vi "校准流程.vi"(0 "校准模式":T3(ring), 5 "参数下拉列表":u16(ring) items=["总氮"=1, "总磷"=2], 7 "测量模式":T1(ring), 9 "量程下拉列表":enum16{"低量程", "高量程"}(ring), 11 "曲线模型":T2={"标液浓度1"=0.0, "测量吸光度1"=0.0, "样品1启用"=FALSE, "标液浓度2"=0.0, "测量吸光度2"=0.0, "样品2启用"=FALSE, "标液浓度3"=0.0, "测量吸光度3"=0.0, "样品3启用"=FALSE, "标液浓度4"=0.0, "测量吸光度4"=0.0, "样品4启用"=FALSE, "标液浓度5"=0.0, "测量吸光度5"=0.0, "样品5启用"=FALSE, "模型"=enum."线性", "精度"=4.0, "XY图"=[], "拟合公式"="", "r^2"=0.0, "标样一校准时间"=timestamp(0 s since 1904-01-01), "标样二校准时间"=timestamp(0 s since 1904-01-01), "标样三校准时间"=timestamp(0 s since 1904-01-01), "标样四校准时间"=timestamp(0 s since 1904-01-01), "标样五校准时间"=timestamp(0 s since 1904-01-01), "二次方程"={"c"=0.0, "x"=0.0, "x^2"=0.0}, "标定时间"=timestamp(0 s since 1904-01-01)} {"标定时间" format="%<%m/%d/%y %H:%M:%S>T"; "标样五校准时间" format="%<%m/%d/%y %H:%M:%S>T"; "标样四校准时间" format="%<%m/%d/%y %H:%M:%S>T"; "标样三校准时间" format="%<%m/%d/%y %H:%M:%S>T"; "标样二校准时间" format="%<%m/%d/%y %H:%M:%S>T"; "标样一校准时间" format="%<%m/%d/%y %H:%M:%S>T"; "r^2" format="%.7f"; "测量吸光度5" format="%#.6f"; "测量吸光度4" format="%#.6f"; "测量吸光度3" format="%#.6f"; "测量吸光度2" format="%#.6f"; "测量吸光度1" format="%#.6f"}) -> ()   [LabVIEW 2016, in "斯坦道CODCr.lvlib"]
panel:
  out "输出簇":cluster{"数据时间":timestamp, "X值":sgl}
  # "校准时间"
  # "标液浓度"
  # "吸光值显示"
  # "标液一"
  # "标液二"
  # "标液三"
  # "零点"
  # "跨度"
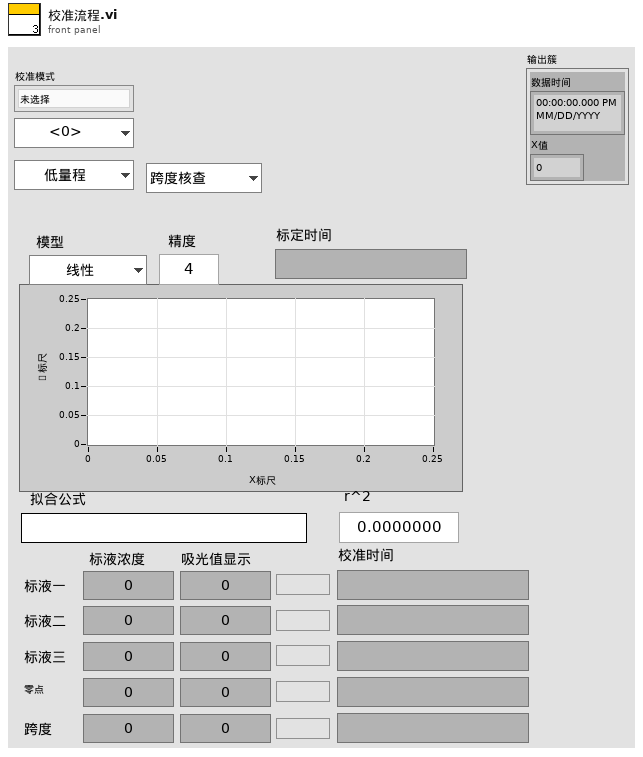
[diagram p1: front panel]
types:
  T1 = enum16{"跨度核查", "水样测量", "零点核查", "标样核查", "加标回收", "快捷测试", "空白校准", "标样校准"}
  T2 = cluster{"标液浓度1":dbl, "测量吸光度1":dbl, "样品1启用":bool, "标液浓度2":dbl, "测量吸光度2":dbl, "样品2启用":bool, "标液浓度3":dbl, "测量吸光度3":dbl, "样品3启用":bool, "标液浓度4":dbl, "测量吸光度4":dbl, "样品4启用":bool, "标液浓度5":dbl, "测量吸光度5":dbl, "样品5启用":bool, "模型":enum32{"线性", "多项式"}, "精度":dbl, "XY图":cluster{"X Values":dbl[], "Y Values":dbl[]}[], "拟合公式":string, "r^2":dbl, "标样一校准时间":timestamp, "标样二校准时间":timestamp, "标样三校准时间":timestamp, "标样四校准时间":timestamp, "标样五校准时间":timestamp, "二次方程":cluster{"c":dbl, "x":dbl, "x^2":dbl}, "标定时间":timestamp}
  T3 = enum32{"未选择", "空白校准", "标样校准", "标样核查", "零点核查", "跨度核查"}
  T4 = enum16{"初始化", "校准启动", "校准运行中", "测试结束", "获取校准数据", "填充校准数据", "流程结束"}
  T5 = cluster{"站号":u16, "量程切换":enum32{"H", "L", "AUTO"}, "控制命令":enum16{"启动测量", "标样核查", "零点核查", "跨度核查", "空白测试", "平行样测试", "加标回收", "空白校准", "标样校准", "初始化（清洗）", "停止测试", "仪器重启", "校时", "模式设置", "测量间隔设置"}, "模式设置":enum16{"待机", "连续模式", "周期模式", "定点模式", "受控模式", "手动模式"}, "测量间隔":u16}
  T6 = enum16{"启动测量", "标样核查", "零点核查", "跨度核查", "空白测试", "平行样测试", "加标回收", "空白校准", "标样校准", "初始化（清洗）", "停止测试", "仪器重启", "校时", "模式设置", "测量间隔设置"}
  T7 = cluster{"因子编码":u32, "单位":u16, "标样参考值":sgl, "水样数据时间":timestamp, "水样实测值":sgl, "水样数据标识":string, "标样数据时间":timestamp, "标样实测值":sgl, "标样数据标识":string, "空白数据时间":timestamp, "空白实测值":sgl, "空白数据标识":string, "零点核查数据时间":timestamp, "零点核查实测值":sgl, "零点核查数据标识":string, "跨度核查数据时间":timestamp, "跨度核查实测值":sgl, "跨度核查数据标识":string, "加标回收数据时间":timestamp, "加标回收实测值":sgl, "加标回收数据标识":string, "平行样数据时间":timestamp, "平行样实测值":sgl, "平行样数据标识":string, "F0":sgl, "F1":sgl, "F2":sgl, "F3":sgl, "F4":sgl, "F5":sgl, "F6":sgl, "F7":sgl, "温度":sgl, "湿度":sgl, "X值":sgl, "fidrange":u16}
  T8 = cluster{"系统时间":timestamp, "工作状态":u16, "测量模式":enum16{"待机", "连续模式", "周期模式", "定点模式", "受控模式", "手动模式"}, "告警代码":u16, "故障代码":u16, "日志代码":u16, "软件版本":u16, "F0":sgl, "F1":sgl, "F2":sgl, "F3":sgl, "T":sgl, "H":sgl, "id":u16, "flowid":u16, "量程":u16, "总磷控温温度1":sgl, "营养盐控温温度2":sgl, "ADC":sgl}
  T9 = cluster{"标液浓度1":dbl, "测量吸光度1":dbl, "样品1启用":bool, "标液浓度2":dbl, "测量吸光度2":dbl, "样品2启用":bool, "标液浓度3":dbl, "测量吸光度3":dbl, "样品3启用":bool, "标液浓度4":dbl, "测量吸光度4":dbl, "样品4启用":bool, "标液浓度5":dbl, "测量吸光度5":dbl, "样品5启用":bool, "模型":enum32{"线性", "多项式"}, "精度":dbl, "XY图":cluster{"X Values":dbl[], "Y Values":dbl[]}[], "拟合公式":string, "r^2":dbl, "标样一校准时间":timestamp, "标样二校准时间":timestamp, "标样三校准时间":timestamp, "标样四校准时间":timestamp, "标样五校准时间":timestamp, "二次方程":cluster{"c":dbl, "x":dbl, "x^2":dbl}, "标定时间":timestamp}[][]
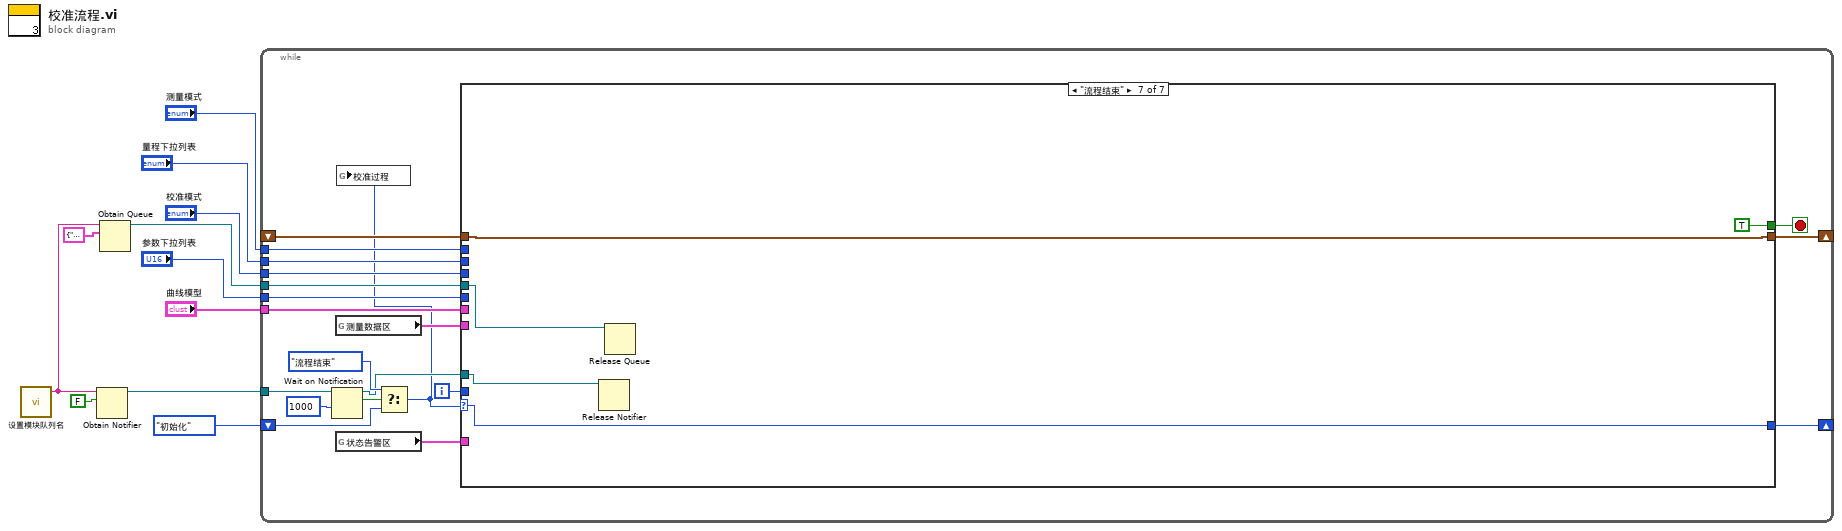
[diagram p0: block diagram]
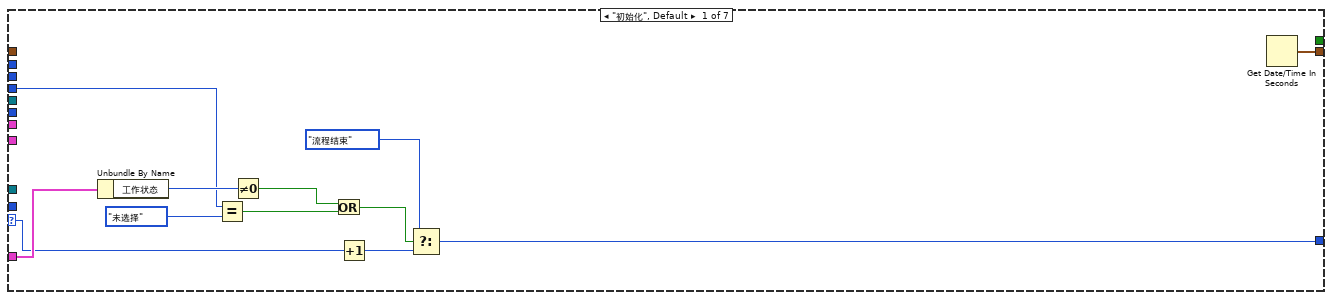
[diagram p2: hidden frame]
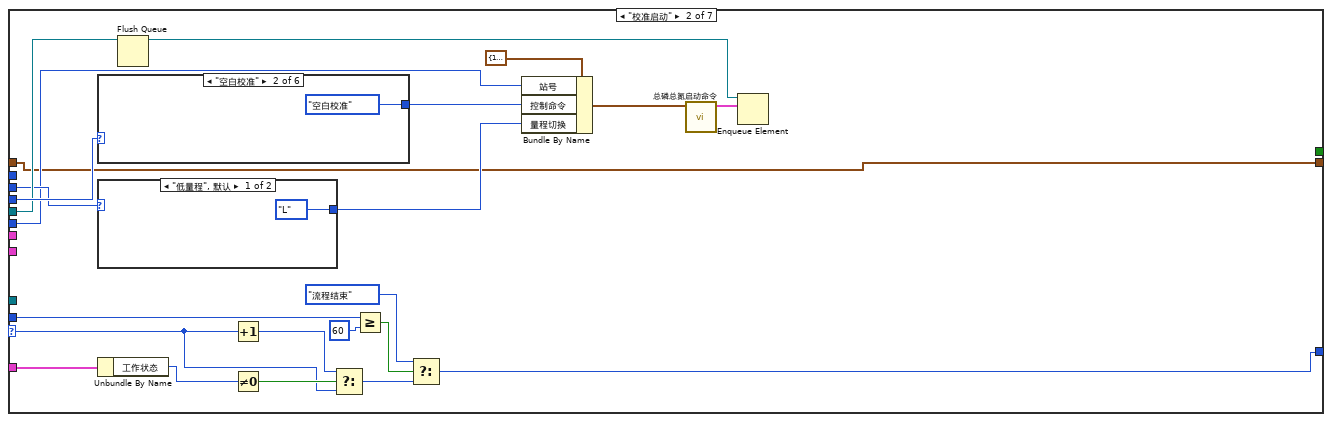
[diagram p3: hidden frame]
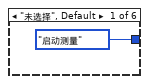
[diagram p4: hidden frame]
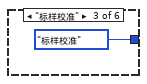
[diagram p5: hidden frame]
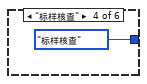
[diagram p6: hidden frame]
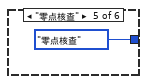
[diagram p7: hidden frame]
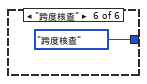
[diagram p8: hidden frame]
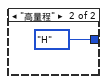
[diagram p9: hidden frame]
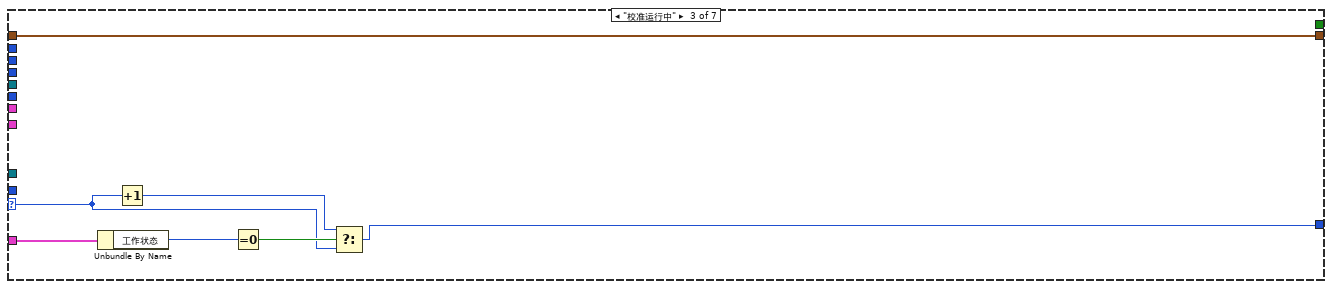
[diagram p10: hidden frame]
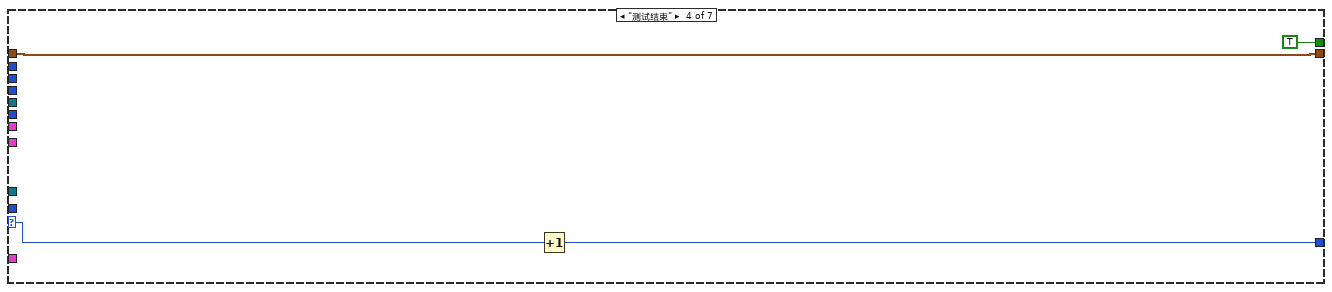
[diagram p11: hidden frame]
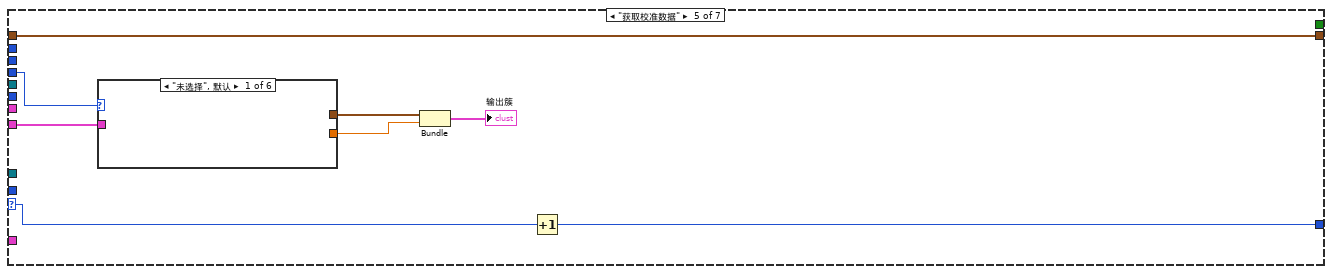
[diagram p12: hidden frame]
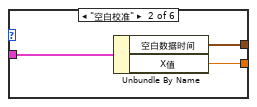
[diagram p13: hidden frame]
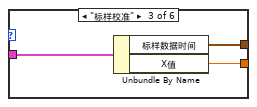
[diagram p14: hidden frame]
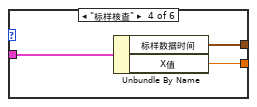
[diagram p15: hidden frame]
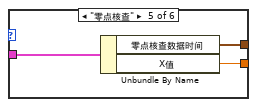
[diagram p16: hidden frame]
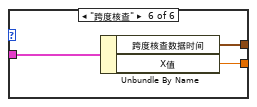
[diagram p17: hidden frame]
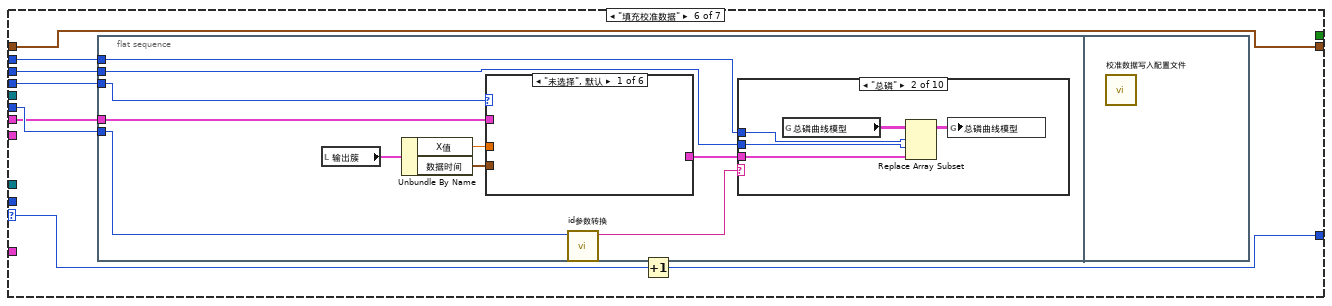
[diagram p18: hidden frame]
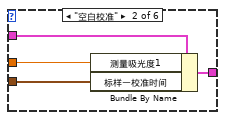
[diagram p19: hidden frame]
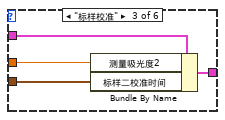
[diagram p20: hidden frame]
diagram:
  n1 = call "设置模块队列名.vi"() -> ("Msg"=w2:string)  [unwired: 5 in]
  n2 = Obtain Notifier(name (unnamed)=w2, notification data type=FALSE) -> (notifier out=w1:refnum<notifier>)  [unwired: 2 in, 2 out]
  n3 = Obtain Queue(name (unnamed)=w2, element data type=cluster{"命令":string, "data":variant} {"命令"="", "data"=variant}) -> (queue out=w8:refnum<queue>)  [unwired: 3 in, 2 out]
  n4 = while {
    tunnel: "校准模式" -> [w30]
    shift-right: [w28] -> _
    shift-left: T4."初始化" ("枚举") -> [w15]
    tunnel: w8 -> [w31]
    tunnel: "量程下拉列表" -> [w27]
    tunnel: "参数下拉列表" -> [w26]
    shift-right: [w25] -> _
    shift-left: _ -> [w24]
    tunnel: "曲线模型" -> [w21]
    tunnel: "测量模式" -> [w20]
    tunnel: w1 -> [w18]
    i -> [w19]
    stop <- w29 stop-if-true
    n5 = Wait on Notification(notifier=w18, timeout in ms (-1)=1000 ("超时毫秒(-1)")) -> (notifier out=w13:refnum<notifier>, notification=w16:bool)  [unwired: 2 in, 2 out]
    n6 = global read "VAR总磷总氮全局变量.vi" "测量数据区"() -> (w23:T7)
    n7 = global read "VAR总磷总氮全局变量.vi" "状态告警区"() -> (w22:T8)
    n8 = Select(t=T4."流程结束", s=w16, f=w15) -> (s? t:f=w12:T4)
    n9 = global write "VAR总磷总氮全局变量.vi" "校准过程"(w12) -> ()
    n10 = case shown="\"流程结束\"" w12 {
      selector: w12 -> [w39 w51 w79 w84 w92 w115 w194]
      tunnel: w31 -> [_ w58 _ _ _ _ w192]
      tunnel: w30 -> [w35 w59 _ _ w89 w109 _]
      tunnel: [_ _ _ TRUE _ _ TRUE] -> w29
      tunnel: [w37 w45 w77 w81 w85 w108 w194] -> w28
      tunnel: w27 -> [_ w57 _ _ _ w112 _]
      tunnel: w26 -> [_ w56 _ _ _ w113 _]
      tunnel: w22 -> [w42 w54 w75 _ _ _ _]
      tunnel: [w43 w55 w76 w83 w91 w114 w193] -> w25
      tunnel: w24 -> [_ w55 w76 w83 w91 w114 w193]
      tunnel: w23 -> [_ _ _ _ w90 _ _]
      tunnel: w21 -> [_ _ _ _ _ w111 _]
      tunnel: w20 -> [_ _ _ _ _ w110 _]
      tunnel: w19 -> [_ w49 _ _ _ _ _]
      tunnel: w13 -> [_ _ _ _ _ _ w191]
      frame "初始化", Default {
        n11 = Unbundle By Name(w42) -> ("工作状态"=w41:u16)
        n12 = Equal?(x=w35, y=T3."未选择") -> (x = y?=w32:bool)
        n13 = Not Equal To 0?(x=w41) -> (x != 0?=w40:bool)
        n14 = Or(x=w40, y=w32) -> (x .or. y?=w33:bool)
        n15 = Increment(x=w39) -> (x+1=w38:T4)
        n16 = Select(t=T4."流程结束", s=w33, f=w38) -> (s? t:f=w37:T4)
        n17 = Get Date/Time In Seconds() -> (seconds since 1Jan1904=w43:timestamp)
      }
      frame "校准启动" {
        n18 = case shown="\"空白校准\"" w59 {
          tunnel: [T6."启动测量" ("控制命令") T6."空白校准" ("控制命令") T6."标样校准" ("控制命令") T6."标样核查" ("控制命令") T6."零点核查" ("控制命令") T6."跨度核查" ("控制命令")] -> w65
          frame "未选择", Default {
          }
          frame "空白校准" {
          }
          frame "标样校准" {
          }
          frame "标样核查" {
          }
          frame "零点核查" {
          }
          frame "跨度核查" {
          }
        }
        n19 = case shown="\"低量程\", 默认" w57 {
          tunnel: [enum32{"H", "L", "AUTO"}."L" ("量程切换") enum32{"H", "L", "AUTO"}."H" ("量程切换")] -> w64
          frame "低量程", Default {
          }
          frame "高量程" {
          }
        }
        n20 = Unbundle By Name(w54) -> ("工作状态"=w53:u16)
        n21 = Flush Queue(queue=w58) -> (queue out=w61:refnum<queue>)  [unwired: 1 in, 2 out]
        n22 = Increment(x=w51) -> (x+1=w50:T4)
        n23 = Not Equal To 0?(x=w53) -> (x != 0?=w52:bool)
        n24 = Select(t=w50, s=w52, f=w51) -> (s? t:f=w46:T4)
        n25 = Greater Or Equal?(x=w49, y=60) -> (x >= y?=w47:bool)
        n26 = Select(t=T4."流程结束", s=w47, f=w46) -> (s? t:f=w45:T4)
        n27 = Bundle By Name(cluster=T5 {"站号"=1, "量程切换"=enum."AUTO", "控制命令"=enum."启动测量", "模式设置"=enum."待机", "测量间隔"=0} ("参数"), "站号"=w56, "控制命令"=w65, "量程切换"=w64) -> (w63:T5)
        n28 = call "总磷总氮启动命令.vi"("参数"=w63) -> ("启动命令"=w60:cluster{"命令":string, "data":variant})  [unwired: 10 in]
        n29 = Enqueue Element(queue=w61, element=w60) -> ()  [unwired: 2 in, 3 out]
      }
      frame "校准运行中" {
        n30 = Unbundle By Name(w75) -> ("工作状态"=w74:u16)
        n31 = Increment(x=w79) -> (x+1=w78:T4)
        n32 = Equal To 0?(x=w74) -> (x = 0?=w80:bool)
        n33 = Select(t=w78, s=w80, f=w79) -> (s? t:f=w77:T4)
      }
      frame "测试结束" {
        n34 = Increment(x=w84) -> (x+1=w81:T4)
      }
      frame "获取校准数据" {
        n35 = case shown="\"未选择\", 默认" w89 {
          tunnel: w90 -> [_ w95 w98 w101 w104 w107]
          tunnel: [_ w94 w97 w100 w103 w106] -> w88
          tunnel: [_ w93 w96 w99 w102 w105] -> w87
          frame "未选择", Default {
          }
          frame "空白校准" {
            n36 = Unbundle By Name(w95) -> ("空白数据时间"=w94:timestamp, "X值"=w93:sgl)
          }
          frame "标样校准" {
            n37 = Unbundle By Name(w98) -> ("标样数据时间"=w97:timestamp, "X值"=w96:sgl)
          }
          frame "标样核查" {
            n38 = Unbundle By Name(w101) -> ("标样数据时间"=w100:timestamp, "X值"=w99:sgl)
          }
          frame "零点核查" {
            n39 = Unbundle By Name(w104) -> ("零点核查数据时间"=w103:timestamp, "X值"=w102:sgl)
          }
          frame "跨度核查" {
            n40 = Unbundle By Name(w107) -> ("跨度核查数据时间"=w106:timestamp, "X值"=w105:sgl)
          }
        }
        n41 = Bundle("跨度核查数据时间"=w88, "X值"=w87) -> (→"输出簇":cluster{"跨度核查数据时间":timestamp, "X值":sgl})  [unwired: 1 in]
        n42 = Increment(x=w92) -> (x+1=w85:T4)
      }
      frame "填充校准数据" {
        n43 = flat-sequence {
          tunnel: w113 -> [w124]
          tunnel: w112 -> [w123]
          tunnel: w111 -> [w122]
          tunnel: w110 -> [w120]
          tunnel: w109 -> [w119]
          frame #0 {
            n44 = local read "输出簇"() -> (w118:cluster{"数据时间":timestamp, "X值":sgl})
            n45 = Unbundle By Name(w118) -> ("X值"=w117:sgl, "数据时间"=w116:timestamp)
            n46 = case shown="\"未选择\", 默认" w119 {
              tunnel: w122 -> [_ w129 w133 w137 w141 w145]
              tunnel: [_ w128 w132 w136 w140 w144] -> w121
              tunnel: w117 -> [_ w127 w131 w135 w139 w143]
              tunnel: w116 -> [_ w126 w130 w134 w138 w142]
              frame "未选择", Default {
              }
              frame "空白校准" {
                n47 = Bundle By Name(cluster=w129, "测量吸光度1"=w127, "标样一校准时间"=w126) -> (w128:T2)
              }
              frame "标样校准" {
                n48 = Bundle By Name(cluster=w133, "测量吸光度2"=w131, "标样二校准时间"=w130) -> (w132:T2)
              }
              frame "标样核查" {
                n49 = Bundle By Name(cluster=w137, "测量吸光度3"=w135, "标样三校准时间"=w134) -> (w136:T2)
              }
              frame "零点核查" {
                n50 = Bundle By Name(cluster=w141, "测量吸光度4"=w139, "标样四校准时间"=w138) -> (w140:T2)
              }
              frame "跨度核查" {
                n51 = Bundle By Name(cluster=w145, "测量吸光度5"=w143, "标样五校准时间"=w142) -> (w144:T2)
              }
            }
            n52 = call "id参数转换.vi"("id"=w124) -> ("table输出"=w125:string)  [unwired: 9 in, 1 out]
            n53 = case shown="\"总磷\"" w125 {
              tunnel: w121 -> [_ w150 w155 w157 w161 w166 w171 w176 w181 w187]
              tunnel: w123 -> [_ w148 w154 w158 w162 w167 w172 w177 w182 w188]
              tunnel: w120 -> [_ w149 w153 w159 w163 w168 w173 w178 w183 w189]
              frame Default {
              }
              frame "总磷" {
                n54 = global read "校准数据全局变量.vi" "总磷曲线模型"() -> (w146:T9)
                n55 = Replace Array Subset(array=w146, new element=w150, index (row)=w149, index (col)=w148) -> (w147:T9)
                n56 = global write "校准数据全局变量.vi" "总磷曲线模型"(w147) -> ()
              }
              frame "总氮" {
                n57 = global read "校准数据全局变量.vi" "总氮曲线模型"() -> (w152:T9)
                n58 = Replace Array Subset(array=w152, new element=w155, index (row)=w153, index (col)=w154) -> (w151:T9)
                n59 = global write "校准数据全局变量.vi" "总氮曲线模型"(w151) -> ()
              }
              frame "氨氮" {
                n60 = global read "校准数据全局变量.vi" "氨氮曲线模型"() -> (w160:T9)
                n61 = Replace Array Subset(array=w160, new element=w157, index (row)=w159, index (col)=w158) -> (w156:T9)
                n62 = global write "校准数据全局变量.vi" "氨氮曲线模型"(w156) -> ()
              }
              frame "磷酸盐" {
                n63 = global read "校准数据全局变量.vi" "磷酸盐曲线模型"() -> (w165:T9)
                n64 = Replace Array Subset(array=w165, new element=w161, index (row)=w163, index (col)=w162) -> (w164:T9)
                n65 = global write "校准数据全局变量.vi" "磷酸盐曲线模型"(w164) -> ()
              }
              frame "硝氮" {
                n66 = global read "校准数据全局变量.vi" "硝氮曲线模型"() -> (w170:T9)
                n67 = Replace Array Subset(array=w170, new element=w166, index (row)=w168, index (col)=w167) -> (w169:T9)
                n68 = global write "校准数据全局变量.vi" "硝氮曲线模型"(w169) -> ()
              }
              frame "亚硝氮" {
                n69 = global read "校准数据全局变量.vi" "亚硝氮曲线模型"() -> (w175:T9)
                n70 = Replace Array Subset(array=w175, new element=w171, index (row)=w173, index (col)=w172) -> (w174:T9)
                n71 = global write "校准数据全局变量.vi" "亚硝氮曲线模型"(w174) -> ()
              }
              frame "硅酸盐" {
                n72 = global read "校准数据全局变量.vi" "硅酸盐曲线模型"() -> (w180:T9)
                n73 = Replace Array Subset(array=w180, new element=w176, index (row)=w178, index (col)=w177) -> (w179:T9)
                n74 = global write "校准数据全局变量.vi" "硅酸盐曲线模型"(w179) -> ()
              }
              frame "硫化物" {
                n75 = global read "校准数据全局变量.vi" "硫化物曲线模型"() -> (w185:T9)
                n76 = Replace Array Subset(array=w185, new element=w181, index (row)=w183, index (col)=w182) -> (w184:T9)
                n77 = global write "校准数据全局变量.vi" "硫化物曲线模型"(w184) -> ()
              }
              frame "CODcr" {
                n78 = global read "校准数据全局变量.vi" "CODcr曲线模型"() -> (w190:T9)
                n79 = Replace Array Subset(array=w190, new element=w187, index (row)=w189, index (col)=w188) -> (w186:T9)
                n80 = global write "校准数据全局变量.vi" "CODcr曲线模型"(w186) -> ()
              }
            }
          }
          frame #1 {
            n81 = call "校准数据写入配置文件.vi"() -> ()  [unwired: 11 in, 1 out]
          }
        }
        n82 = Increment(x=w115) -> (x+1=w108:T4)
      }
      frame "流程结束" {
        n83 = Release Notifier(notifier=w191) -> ()  [unwired: 2 in, 3 out]
        n84 = Release Queue(queue=w192) -> ()  [unwired: 2 in, 3 out]
      }
    }
  }
